vi "Read Register (float).vi"(0 "Refnum in":refnum<visa-resource-name>, 1 "startReg":u16, 5 "Mode":T1, 7 "WordCount":u16=2, 9 "Register type":enum16{"Input", "Holding"}(ring), 11 "error in (no error)":errorcluster, 12 "Enable":bool) -> (4 "Refnum Out":refnum<visa-resource-name>, 6 "ModeOut":T1, 8 "Data":sgl[](array[numeric]), 10 "first element":sgl, 15 "error out":errorcluster)   [LabVIEW 2020]
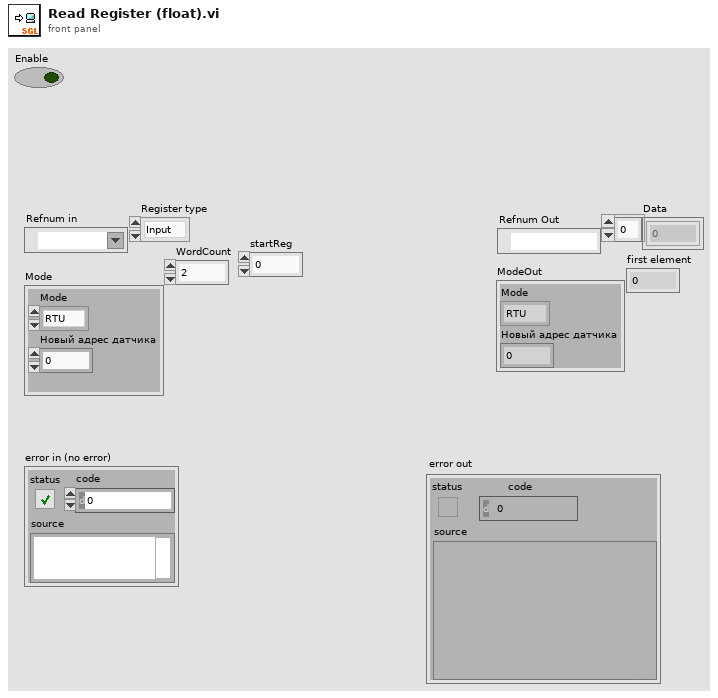
[diagram p1: front panel]
types:
  T1 = cluster{"Mode":enum16{"RTU", "ASCII"}, "Новый адрес датчика":u16}
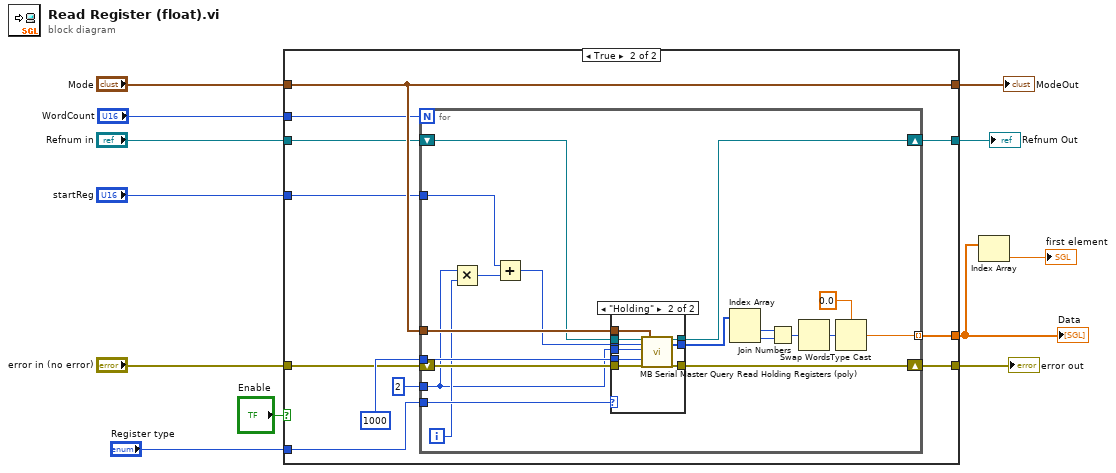
[diagram p0: block diagram]
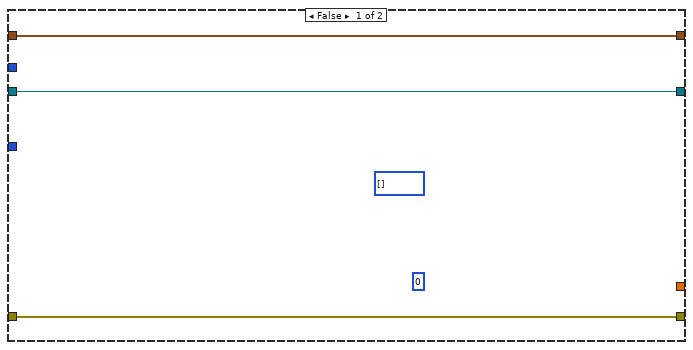
[diagram p2: hidden frame]
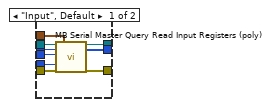
[diagram p3: hidden frame]
diagram:
  n1 = case shown="True" "Enable" {
    tunnel: "Mode" -> [w14 w23]
    tunnel: "error in (no error)" -> [w15 w25]
    tunnel: "Refnum in" -> [w13 w22]
    tunnel: "startReg" -> [_ w16]
    tunnel: "WordCount" -> [_ w18]
    tunnel: [w15 w24] -> w9
    tunnel: [w14 w23] -> w7
    tunnel: [w13 w21] -> w6
    tunnel: "Register type" -> [_ w20]
    tunnel: [_ w19] -> w2
    frame False {
      (unwired) u16[] [] ("Holding Registers")
      (unwired) u16 0 ("Numeric")
    }
    frame True {
      n2 = for {
        N: w18 -> [_]
        tunnel: u32 1000 ("Timeout") -> [w45]
        tunnel: w23 -> [w42]
        tunnel: w20 -> [w38]
        tunnel: [w32] -> w19 mode=indexing
        shift-right: [w43] -> w24
        shift-left: w25 -> [w44]
        shift-right: [w40] -> w21
        shift-left: w22 -> [w41]
        tunnel: u16 2 ("Quantity") -> [w30]
        tunnel: w16 -> [w28]
        i -> [w31]
        n3 = Multiply(x=w30, y=w31) -> (x*y=w29:i32)
        n4 = Add(x=w28, y=w29) -> (x+y=w27:i32)
        n5 = case shown="\"Holding\"" w38 {
          tunnel: w45 -> [w49 w63]
          tunnel: w44 -> [w48 w62]
          tunnel: w27 -> [w51 w61]
          tunnel: [w47 w60] -> w43
          tunnel: w42 -> [w54 w59]
          tunnel: w41 -> [w52 w58]
          tunnel: [w53 w57] -> w40
          tunnel: w30 -> [w50 w56]
          tunnel: [w46 w55] -> w39
          frame "Input", Default {
            n6 = call <vilib>:"MB Serial Master Query Read Input Registers (poly).vi"("VISA resource name"=w52, "Starting Address"=w51, "Quantity"=w50, "Timeout"=w49, "error in"=w48, "Serial Parameters"=w54) -> ("VISA resource name out"=w53:refnum<visa-resource-name>, "Input Registers"=w46:u16[], "error out"=w47:errorcluster)  [unwired: 10 in, 1 out]
          }
          frame "Holding" {
            n7 = call <vilib>:"MB Serial Master Query Read Holding Registers (poly).vi"("VISA resource name"=w58, "Starting Address"=w61, "Quantity"=w56, "Timeout"=w63, "error in"=w62, "Serial Parameters"=w59) -> ("VISA resource name out"=w57:refnum<visa-resource-name>, "Holding Registers"=w55:u16[], "error out"=w60:errorcluster)  [unwired: 10 in, 1 out]
          }
        }
        n8 = Index Array(array=w39) -> (element #1=w35:u16, element #2=w33:u16)  [unwired: 2 in]
        n9 = Join Numbers(hi=w35, lo=w33) -> ((hi.lo)=w37:u32)
        n10 = Swap Words(1:w37) -> (0:w36:u32)
        n11 = Type Cast(type=sgl 0.0 ("p_atm"), x=w36) -> (*(type *) &x=w32:sgl)
      }
    }
  }
  "error out" <- w9
  "ModeOut" <- w7
  "Refnum Out" <- w6
  "Data" <- w2
  n12 = Index Array(array=w2) -> (element=→"first element":sgl)  [unwired: 1 in]
